vi "decimate-value_single_axis.vi"(7 "type":T1, 8 "error in (no error)":errorcluster, 9 "interval":dbl format="%#_13g", 10 "y_axis in":dbl[](array[numeric]), 11 "x_axis in":dbl[](array[numeric])) -> (0 "error out":errorcluster, 2 "y_axis out":dbl[](array[numeric]), 3 "x_axis out":dbl[](array[numeric]))   [LabVIEW 2015, in "lv-graph.lvlib"]
doc: "This VI will decimate a given dataset, following the rule that you can display, at most two points per pixel per plot. If the number of points exceeds the number of pixels (wired from height_width). For decimation, it'll group equal sets of points (except the last set) for data representation. As configured, the way the points are represented can be configured as follows: (1) average: this will get the mean of the points per group (2) min_max will average the min/max values for the group (3) max: will return the max value, (4) min: will return the min value, (5) first will return the first value and (6) last will return the last value."
uses:
  lv-graph.lvlib
  _controls/decimation_type.ctl
  <vilib>/Analysis/baseanly.llb/Mean (DBL).vi
  <vilib>/Analysis/NI_AALBase.lvlib
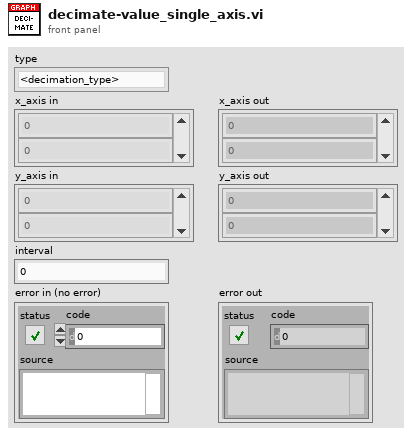
[diagram p1: front panel]
types:
  T1 = typedef "lv-graph.lvlib/decimation_type.ctl" = enum16{"<decimation_type>", "average", "min_max", "max", "min", "first", "last"}
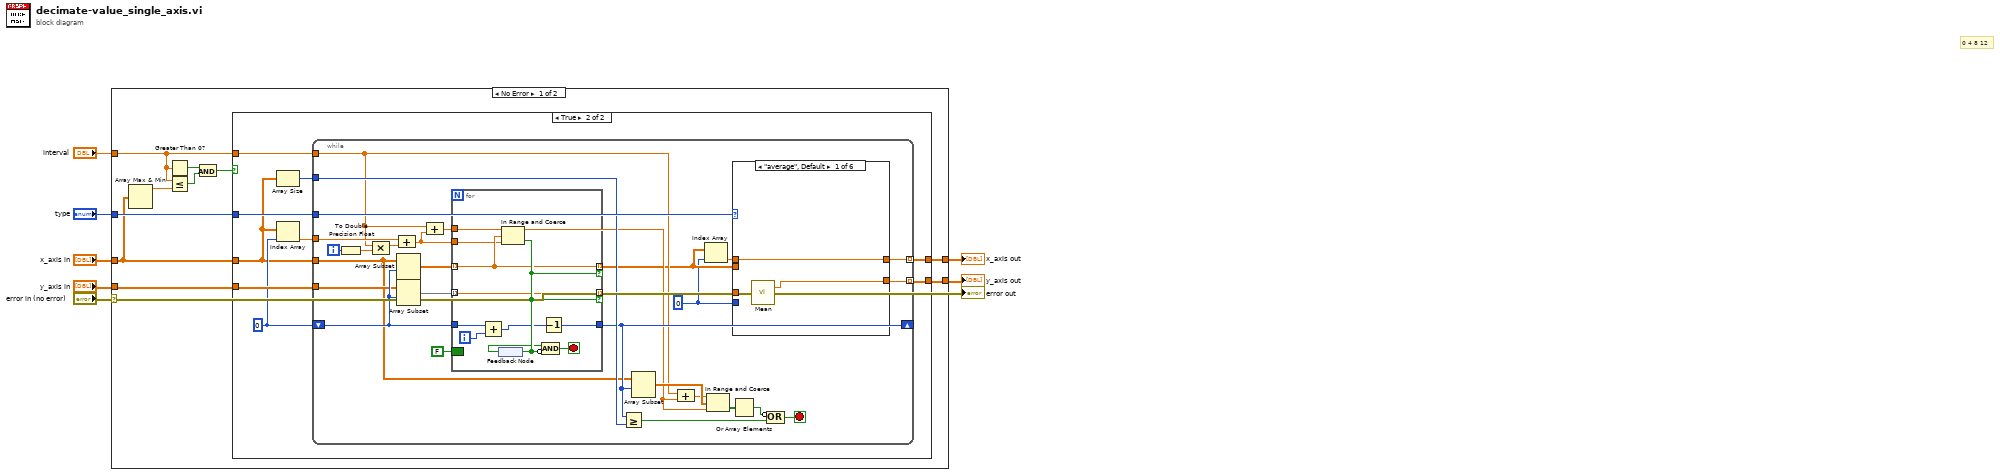
[diagram p0: block diagram]
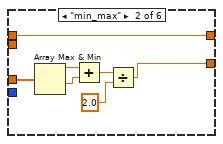
[diagram p3: hidden frame]
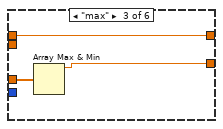
[diagram p4: hidden frame]
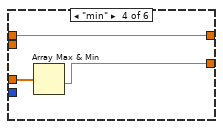
[diagram p5: hidden frame]
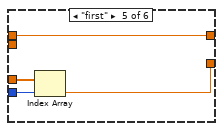
[diagram p6: hidden frame]
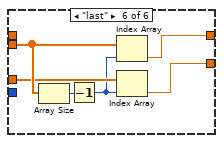
[diagram p7: hidden frame]
diagram:
  # "0 4 8 12"
  n1 = case shown="No Error" "error in (no error)" {
    tunnel: "x_axis in" -> [w10 _]
    tunnel: "y_axis in" -> [w14 _]
    tunnel: "type" -> [w17 _]
    tunnel: [w16 _] -> w4
    tunnel: [w15 _] -> w3
    tunnel: "interval" -> [w9 _]
    frame No Error {
      n2 = Array Max & Min(array=w10) -> (max value=w12:dbl)  [unwired: 3 out]
      n3 = Greater Than 0?(x=w9) -> (x > 0?=w13:bool)
      n4 = Less Or Equal?(x=w9, y=w12) -> (x <= y?=w11:bool)
      n5 = And(x=w13, y=w11) -> (x .and. y?=w8:bool)
      n6 = case shown="True" w8 {
        tunnel: w10 -> [w19 w21]
        tunnel: w14 -> [w18 w25]
        tunnel: w17 -> [_ w28]
        tunnel: [w19 w27] -> w16
        tunnel: [w18 w26] -> w15
        tunnel: w9 -> [_ w24]
        frame False {
        }
        frame True {
          w22 = 0
          n7 = Array Size(array=w21) -> (size(s)=w20:i32)
          n8 = Index Array(array=w21, index=w22) -> (element=w23:dbl)
          n9 = while {
            tunnel: w28 -> [w54]
            tunnel: [w56] -> w26 mode=indexing
            tunnel: [w55] -> w27 mode=indexing
            tunnel: w21 -> [w43]
            tunnel: w25 -> [w48]
            shift-right: [w47] -> _
            shift-left: w22 -> [w50]
            tunnel: w24 -> [w35]
            tunnel: w20 -> [w49]
            tunnel: w23 -> [w39]
            i -> [w36]
            stop <- w33 stop-if-true
            w31 = 0 ("index")
            n10 = To Double Precision Float(number=w36) -> (double precision float=w42:dbl)
            n11 = Compound Arithmetic op=MULTIPLY(w35, w42) -> (w40:dbl)
            n12 = Array Subset(array=w43, index=w50) -> (w52:dbl[])  [unwired: 1 in]
            n13 = Array Subset(array=w48, index=w50) -> (w51:dbl[])  [unwired: 1 in]
            n14 = Compound Arithmetic op=ADD(w39, w40) -> (w38:dbl)
            n15 = Compound Arithmetic op=ADD(w35, w38) -> (w37:dbl)
            n16 = for {
              tunnel: w50 -> [w67]
              tunnel: [w57] -> w47
              tunnel: w52 -> [w62] mode=indexing
              tunnel: w51 -> [w61] mode=indexing
              tunnel: [w62] -> w32 mode=indexing if=w65
              tunnel: [w61] -> w53 mode=indexing if=w65
              tunnel: w38 -> [w59]
              tunnel: w37 -> [w58]
              border: FALSE -> [_]
              i -> [w66]
              stop <- w60 stop-if-true
              n17 = Add(x=w67, y=w66) -> (x+y=w63:i32)
              n18 = feedback #1() -> (w64:bool)
              n19 = In Range and Coerce(upper limit=w58, x=w62, lower limit=w59) -> (In Range?=w65:bool)  [unwired: 1 out]
              n20 = feedback-in #1(w65) -> ()
              n21 = Decrement(x=w63) -> (x-1=w57:i32)
              n22 = Compound Arithmetic op=AND(w64, invert w65) -> (w60:bool)
            }
            n23 = Greater Or Equal?(x=w47, y=w49) -> (x >= y?=w34:bool)
            n24 = Array Subset(array=w43, index=w47) -> (w46:dbl[])  [unwired: 1 in]
            n25 = Compound Arithmetic op=ADD(w35, w37) -> (w41:dbl)
            n26 = Index Array(array=w32, index=w31) -> (element=w30:dbl)
            n27 = In Range and Coerce(upper limit=w41, x=w46, lower limit=w37) -> (In Range?=w45:bool[])  [unwired: 1 out]
            n28 = case shown="\"average\", Default" w54 {
              tunnel: w32 -> [_ _ _ _ _ w91]
              tunnel: w53 -> [w70 w77 w80 w83 w87 w89]
              tunnel: [w69 w76 w79 w82 w86 w92] -> w56
              tunnel: [w68 w71 w78 w81 w84 w93] -> w55
              tunnel: w31 -> [_ _ _ _ w85 _]
              tunnel: w30 -> [w68 w71 w78 w81 w84 _]
              frame "average", Default {
                n29 = call-poly <vilib>:"Mean.vi"("X"=w70) -> ("mean"=w69:dbl)  [unwired: 1 out]
              }
              frame "min_max" {
                n30 = Array Max & Min(array=w77) -> (max value=w75:dbl, min value=w74:dbl)  [unwired: 2 out]
                n31 = Add(x=w75, y=w74) -> (x+y=w73:dbl)
                n32 = Divide(x=w73, y=2.0) -> (x/y=w76:dbl)
              }
              frame "max" {
                n33 = Array Max & Min(array=w80) -> (max value=w79:dbl)  [unwired: 3 out]
              }
              frame "min" {
                n34 = Array Max & Min(array=w83) -> (min value=w82:dbl)  [unwired: 3 out]
              }
              frame "first" {
                n35 = Index Array(array=w87, index=w85) -> (element=w86:dbl)
              }
              frame "last" {
                n36 = Array Size(array=w91) -> (size(s)=w90:i32)
                n37 = Decrement(x=w90) -> (x-1=w88:i32)
                n38 = Index Array(array=w91, index=w88) -> (element=w93:dbl)
                n39 = Index Array(array=w89, index=w88) -> (element=w92:dbl)
              }
            }
            n40 = Or Array Elements(Boolean array=w45) -> (logical OR=w44:bool)
            n41 = Compound Arithmetic op=OR(invert w44, w34) -> (w33:bool)
          }
        }
      }
    }
    frame Error {
    }
  }
  "x_axis out" <- w4
  "y_axis out" <- w3
  "error out" <- "error in (no error)"
